vi "ctl.vi"(6 "heater":string, 7 "LVWSR":refnum<class "Web Request.lvclass">, 8 "d":dbl, 9 "i":dbl, 10 "p":dbl, 11 "instr":string) -> ()   [LabVIEW 2017]
uses:
  <vilib>/wsapi/Web Request.lvclass
  Controller/Messages/Change Heater Ctl Params MSG/Change Heater Ctl Params.lvclass
  C:/Program Files (x86)/National Instruments/LabVIEW 2017/vi.lib/ActorFramework/Message/Message.lvclass
  Controller/Messages/Change Heater Ctl Params MSG/Change Heater Ctl Params.lvclass/Change Heater Ctl Params.ctl
  <vilib>/ActorFramework/Message Enqueuer/Message Enqueuer.lvclass/Message Enqueuer.ctl
  Controller/Messages/Change Heater Ctl Params MSG/Write id.vi
  <vilib>/ActorFramework/Message Priority Queue/Priority Enqueue.vi
  Controller/gController.lvclass
  <vilib>/ActorFramework/Message Enqueuer/Message Enqueuer.lvclass
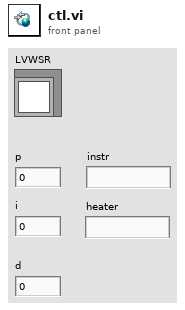
[diagram p1: front panel]
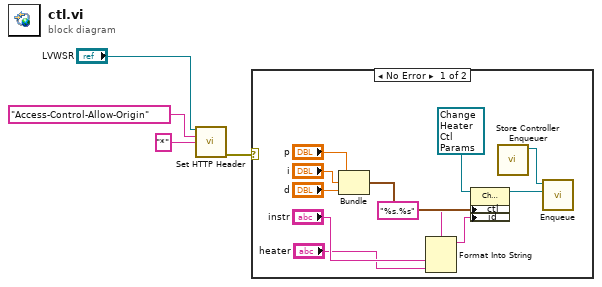
[diagram p0: block diagram]
diagram:
  n1 = call <vilib>:"Set HTTP Header.vi"("LabVIEW Web Service Request"="LVWSR", "header"="Access-Control-Allow-Origin", "header value"="*") -> ("error out"=w1:errorcluster)  [unwired: 11 in, 1 out]
  n2 = case shown="No Error" w1 {
    frame No Error {
      n3 = Bundle("p"="p", "i"="i", "d"="d") -> (w10:cluster{"p":dbl, "i":dbl, "d":dbl})  [unwired: 1 in]
      n4 = Format Into String(format string="%s.%s", "instr", "heater") -> (resulting string=w8:string)  [unwired: 2 in, 1 out]
      n5 = property class="Change Heater Ctl Params"(reference=refnum<class "Change Heater Ctl Params.lvclass"> refnum ("Controller.lvlib:Change Heater Ctl Params.lvclass"), "ctl"=w10, "id"=w8) -> (reference out=w9:refnum<class "Change Heater Ctl Params.lvclass">)  [unwired: 1 in, 1 out]
      n6 = call "Store Controller Enqueuer.vi"() -> ("Controller Enqueuer Out"=w15:refnum<class "Message Enqueuer.lvclass">)  [unwired: 11 in]
      n7 = call <vilib>:"Enqueue.vi"("Message"=w9, "Message Enqueuer in"=w15) -> ()  [unwired: 8 in, 2 out]
    }
    frame Error {
    }
  }
